vi "Clamping.vi"(0 "Source Image":T3, 2 "ROI Descriptor":T2 {"Contours"."Type" items=["No Selection", "Point", "Line", "Rectangle", "Oval", "Polygon", "Freehand Region", "Annulus", "Unused2", "Unused3", "Broken Line", "Freehand Line", "Rotated Rectangle"]}) -> (7 "Image Out":T3, 9 "Clamp Results":T8)   [LabVIEW 2015]
uses:
  <vilib>/vision/Pattern Matching.llb/IMAQ Curve Parameters.ctl
  <vilib>/vision/Clamp.llb/Edge Polarity Type.ctl
  <vilib>/vision/Image Controls.llb/IMAQ Image.ctl
  <vilib>/vision/NI_Vision_Development_Module.lvlib
panel:
  in  "Coordinate System":T1 {"Measurement System"."Axis Reference" items=["Direct", "Indirect"]; "Measurement System"."Angle (deg)" format="%.2f"; "Measurement System"."Origin"."Y" format="%.2f"; "Measurement System"."Origin"."X" format="%.2f"; "Reference System"."Axis Reference" items=["Direct", "Indirect"]; "Reference System"."Angle (deg)" format="%.2f"; "Reference System"."Origin"."Y" format="%.2f"; "Reference System"."Origin"."X" format="%.2f"}
  in  "Overlay Settings":T4={"Show Search Area"=FALSE, "Show Curves"=FALSE, "Show Clamp Locations"=FALSE, "Show Result"=TRUE, "Search Area Color"=6618880, "Curves Color"=12764, "Clamp Locations Color"=16776960, "Result Color"=16711680, "Overlay Group Name"=""}
  in  "Clamp Settings":T6={"Angle Range (+/-)"=5.0, "Edge Polarity"={"Start"=0, "End"=0}} {"Edge Polarity"."End" items=["Any", "Rising", "Falling"]; "Edge Polarity"."Start" items=["Any", "Rising", "Falling"]}
  in  "Curve Extraction Settings":T7={"Extraction Mode"=0, "Edge Threshold"=75, "Edge Filter Size"=0, "Min Length"=10, "Row Search Step Size"=10, "Col Search Step Size"=10, "Max Endpoint Gap"=5, "Closed"=FALSE, "Subpixel"=FALSE} {"Extraction Mode" items=["Normal", "Uniform Regions"]; "Edge Filter Size" items=["Fine", "Normal", "Contour Tracing"]; "Max Endpoint Gap" min=0; "Col Search Step Size" min=1 max=255 step=1; "Row Search Step Size" min=1 max=255 step=1; "Min Length" min=0; "Edge Threshold" min=1 max=350 step=1}
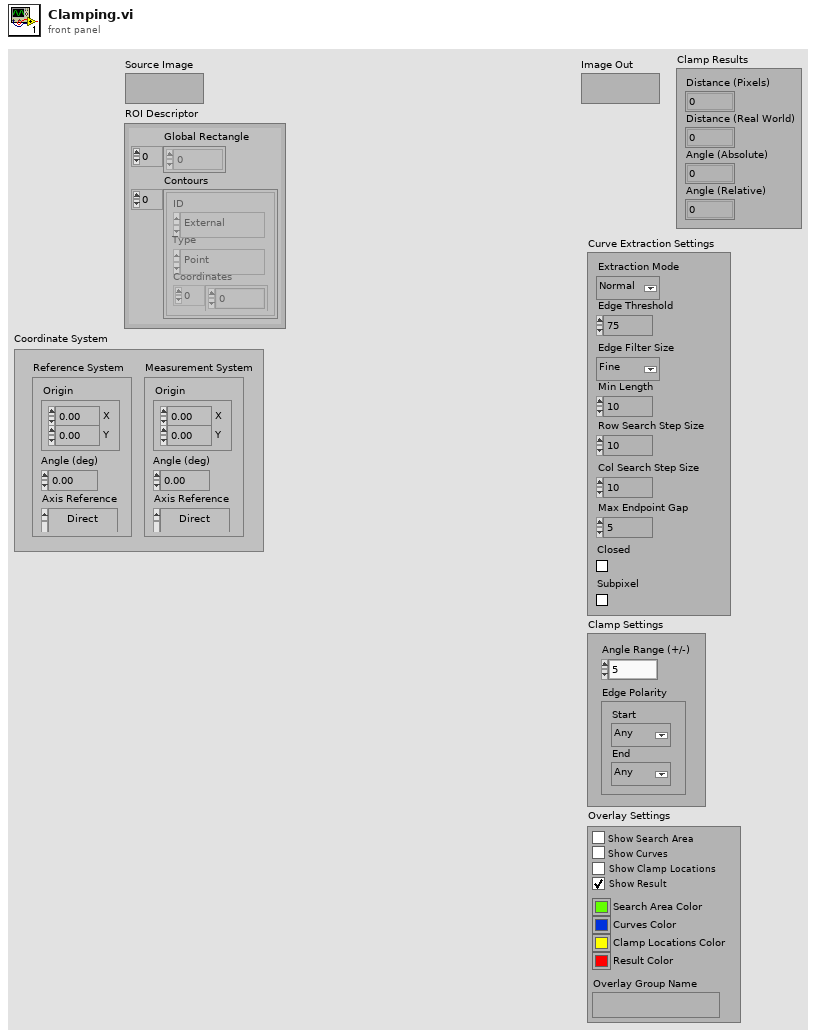
[diagram p1: front panel]
types:
  T1 = typedef "IMAQ Coordinate System" = cluster{"Reference System":cluster{"Origin":cluster{"X":sgl, "Y":sgl}, "Angle (deg)":sgl, "Axis Reference":u32}, "Measurement System":cluster{"Origin":cluster{"X":sgl, "Y":sgl}, "Angle (deg)":sgl, "Axis Reference":u32}}
  T2 = typedef "ROI Descriptor" = cluster{"Global Rectangle":i32[], "Contours":cluster{"ID":enum32{"External", "Internal"}, "Type":u32, "Coordinates":i32[]}[]}
  T3 = typedef "IMAQ Image.ctl" = refnum<image>
  T4 = cluster{"Show Search Area":bool, "Show Curves":bool, "Show Clamp Locations":bool, "Show Result":bool, "Search Area Color":u32, "Curves Color":u32, "Clamp Locations Color":u32, "Result Color":u32, "Overlay Group Name":string}
  T5 = typedef "Edge Polarity Type.ctl" = u32
  T6 = cluster{"Angle Range (+/-)":dbl, "Edge Polarity":cluster{"Start":T5, "End":T5}}
  T7 = typedef "IMAQ Curve Parameters.ctl" = cluster{"Extraction Mode":u32, "Edge Threshold":i32, "Edge Filter Size":u32, "Min Length":i32, "Row Search Step Size":i32, "Col Search Step Size":i32, "Max Endpoint Gap":i32, "Closed":bool, "Subpixel":bool}
  T8 = cluster{"Distance (Pixels)":dbl, "Distance (Real World)":dbl, "Angle (Absolute)":dbl, "Angle (Relative)":dbl}
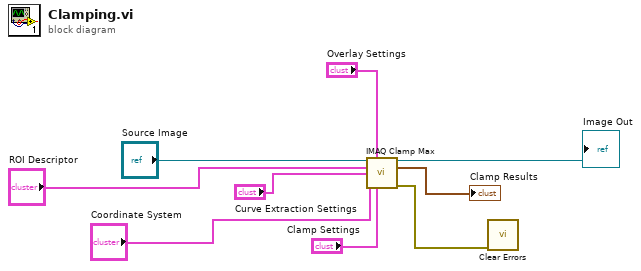
[diagram p0: block diagram]
diagram:
  n1 = call "IMAQ Clamp Max"("Source Image"="Source Image", "Overlay Settings"="Overlay Settings", "ROI Descriptor"="ROI Descriptor", "Curve Extraction Settings"="Curve Extraction Settings", "Coordinate System"="Coordinate System", "Clamp Settings"="Clamp Settings") -> ("Image Out"=→"Image Out":T3, "Clamp Results"=→"Clamp Results":T8, "error out"=w5:errorcluster)  [unwired: 4 in, 3 out]
  n2 = call <vilib>:"Clear Errors.vi"("error in (no error)"=w5) -> ()  [unwired: 5 in, 2 out]
